vi "InstrumentSetup.vi"() -> ()   [LabVIEW 2019, in "InstrControl.lvclass"]
uses:
  InstrControl.lvclass
  SupplyControl/Keithley 236 & 237/KE236.lvclass
  SupplyControl/Keithley 6517/KE6517.lvclass
  SupplyControl/Keithley 2410/KE2410.lvclass
  SupplyControl/Keithley 487/KE487.lvclass
  ArduinoControl/ArduinoControl.lvclass
  MultimeterControl/Keithley 2000/KE2000.lvclass
  LCRControl/WK6440B/WK6440B.lvclass
  Switching/Pickering/Pickering.lvclass
  LCRControl/WK6425/WK6425.lvclass
  Switching/Keithley 3706A/KE3706A.lvclass
  Switching/LXIPXISwitching/LXIPXISwitching.lvclass
panel:
  in  "LXI/PXI Configurations":T1={"MUX"="1", "Matrix"="4", "Breadboard"="5", "LXIPXI Switching"=refnum, "MUX PN"="40-635-108", "Matrix  PN"="40-332-002", "Breadboard PN"="40-220A-501-S6", "MUX ID"="1", "Matrix ID"="4", "Breadboard ID"="5"}
  in  "Keithley 3706A Configurations":T2={"Mux1 slot"="1", "Mux2 slot"="2", "KE3706A"=refnum}
  in  "Keithley 487_2 Configurations":T3 {"Range:" items=["Autorange", "2nA", "20nA", "200nA", "2 microAmp", "20 microAmp", "200 microAmp", "2 milliAmp"]; "Compliance" items=["20µA", "2mA"]}
  in  "Instrument addresses":T4={"KE 2410"={"Instrument name"="Keithley 2410", "address"="GPIB0::16::INSTR", "Instrument type"=0}, "KE 6517"={"Instrument name"="Keithley 6517", "address"="", "Instrument type"=0}, "KE 487"={"Instrument name"="Keithley 487", "address"="", "Instrument type"=0}, "KE 236"={"Instrument name"="Keithley 236", "address"="", "Instrument type"=0}, "WK 6440B"={"Instrument name"="WayneKerr 6440B", "address"="GPIB0::6::INSTR", "Instrument type"=1}, "WK 6425"={"Instrument name"="WayneKerr 6425", "address"="", "Instrument type"=1}, "Pickering Matrix"={"Instrument name"="Pickering Matrix", "address"="GPIB0::10::INSTR", "Instrument type"=3}, "KE 2000"={"Instrument name"="Keithley 2000", "address"="GPIB0::19::INSTR", "Instrument type"=2}, "KE3706A Switching"={"Instrument name"="KE3706A", "address"="GPIB0::11::INSTR", "Instrument type"=3}} {"KE3706A Switching"."Instrument type" items=["Supply", "LCR", "Multimeter", "Switching"]; "KE 2000"."Instrument type" items=["Supply", "LCR", "Multimeter", "Switching"]; "Pickering Matrix"."Instrument type" items=["Supply", "LCR", "Multimeter", "Switching"]; "WK 6425"."Instrument type" items=["Supply", "LCR", "Multimeter", "Switching"]; "WK 6440B"."Instrument type" items=["Supply", "LCR", "Multimeter", "Switching"]; "KE 236"."Instrument type" items=["Supply", "LCR", "Multimeter", "Switching"]; "KE 487"."Instrument type" items=["Supply", "LCR", "Multimeter", "Switching"]; "KE 6517"."Instrument type" items=["Supply", "LCR", "Multimeter", "Switching"]; "KE 2410"."Instrument type" items=["Supply", "LCR", "Multimeter", "Switching"]}
  in  "WayneKerr 6425 Configurations":T5={"RC Configuration"=0, "AC amplitude [V]"=0.1, "AC frequency [Hz]"=1000, "WK6425"=refnum} {"RC Configuration" items=["serial", "parallel"]}
  in  "Pickering MUX & Matrix Configurations":T6={"Matrix address"="1", "Mux1 address"="4", "Mux2 address"="5", "Pickering"=refnum, "Matrix X Channels"={"Bias Supply / SMU LO"=5, "Bias Supply / SMU HI"=6, "CV Box LO"=3, "CV Box HI"=4, "CV Box LO IN"=7, "CV Box HI IN"=8, "Volt meter LO"=1, "Volt meter HI"=2, "Mux1 C1"=9, "Mux1 C2"=10, "Mux2 C1"=11, "Mux2 C2"=12}}
  in  "WayneKerr 6440B Configurations":T7={"RC Configuration"=0, "AC amplitude [V]"=0.1, "AC frequency [Hz]"=1000, "WK6440B"=refnum} {"RC Configuration" items=["serial", "parallel"]}
  in  "Keithley 2000 Configurations":T8={"Range"=0, "Range Value"=100.0, "Function"=3, "KE2000"=refnum} {"Function" items=["AC Current", "DC Current", "AC Voltage", "DC Voltage", "2W-Resistance", "4W-Resistance", "Period", "Frequency", "Temperature", "Diode", "Continuity"]; "Range Value" format="%#.2g"; "Range" items=["Auto", "Manual"]}
  in  "Arduino Configuration":T9={"VISA address"="COM24", "T sensor"=enum."SHT", "Arduino"=refnum}
  in  "Keithley 487 Configurations":T3 {"Range:" items=["Autorange", "2nA", "20nA", "200nA", "2 microAmp", "20 microAmp", "200 microAmp", "2 milliAmp"]; "Compliance" items=["20µA", "2mA"]}
  in  "Keithley 2410 Configurations":T10={"Current Limit"=0.0001, "KE2410"=refnum}
  in  "Keithley 6517 Configurations":T11={"Current Limit"=1, "KE6517"=refnum} {"Current Limit" items=["OFF", "ON"]}
  in  "Keithley 236 Configurations":T12={"current \ncompliance level"=0.0001, "compliance/\nmeasurement range (auto:0)"=6, "KE236"=refnum} {"compliance/\nmeasurement range (auto:0)" items=["auto / auto", "1 nA / 1.1 V", "10 nA / 11 V", "100 nA / 110 V", "0.001 mA / 110 V", "0.01 mA / 110 V", "0.1 mA / 110 V", "1 mA / 110 V", "10 mA / 110 V", "100 mA / 110 V"]; "current \ncompliance level" format="%.4f"}
  in  "Default GPIB addresses":T13={"KE 487"="22", "KE 6517"="27", "WK 6425"="17", "KE 236"="16", "HP 4263B"="18", "KE 2000"="19", "KE 2410"="24", "WK 6440B"="23", "Matrix"="10"}
  # "PROPERTY CLUSTERS + DEFAULT VALUES FOR INSTRUMENT SETUP"
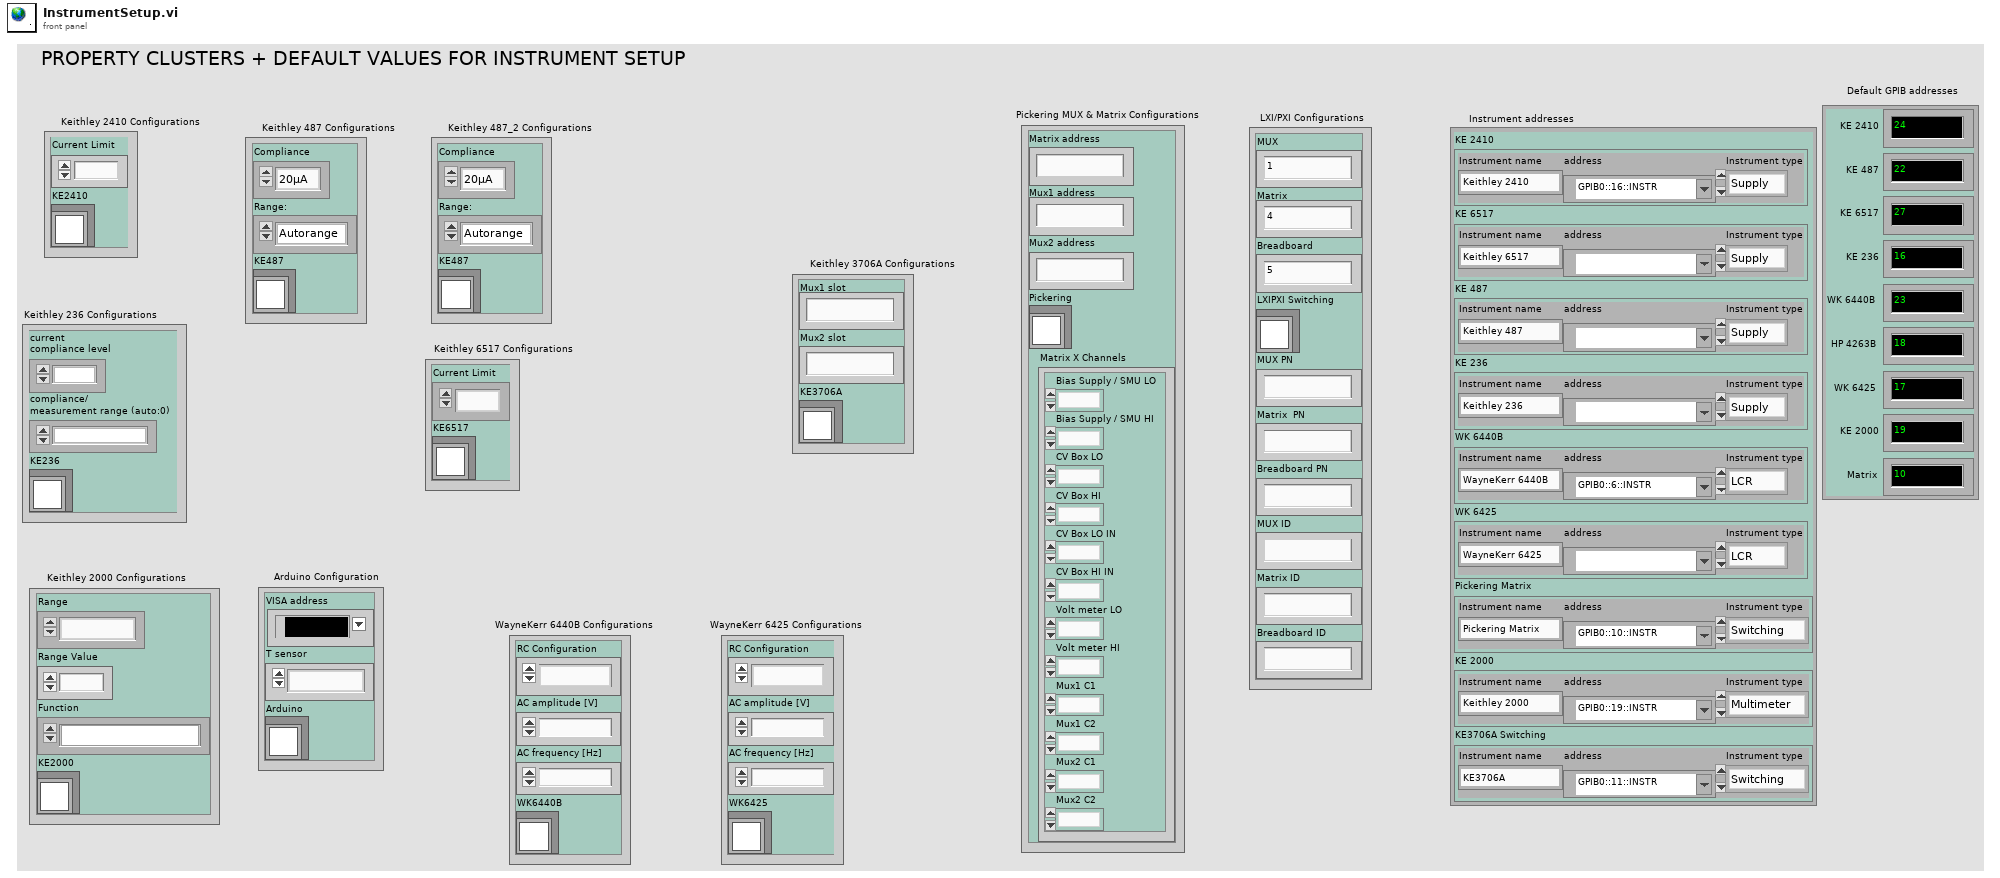
[diagram p1: front panel]
types:
  T1 = cluster{"MUX":string, "Matrix":string, "Breadboard":string, "LXIPXI Switching":refnum<class "LXIPXISwitching.lvclass">, "MUX PN":string, "Matrix  PN":string, "Breadboard PN":string, "MUX ID":string, "Matrix ID":string, "Breadboard ID":string}
  T2 = cluster{"Mux1 slot":string, "Mux2 slot":string, "KE3706A":refnum<class "KE3706A.lvclass">}
  T3 = cluster{"Compliance":u16, "Range:":u16, "KE487":refnum<class "KE487.lvclass">}
  T4 = cluster{"KE 2410":cluster{"Instrument name":string, "address":refnum<visa-resource-name>, "Instrument type":u16}, "KE 6517":cluster{"Instrument name":string, "address":refnum<visa-resource-name>, "Instrument type":u16}, "KE 487":cluster{"Instrument name":string, "address":refnum<visa-resource-name>, "Instrument type":u16}, "KE 236":cluster{"Instrument name":string, "address":refnum<visa-resource-name>, "Instrument type":u16}, "WK 6440B":cluster{"Instrument name":string, "address":refnum<visa-resource-name>, "Instrument type":u16}, "WK 6425":cluster{"Instrument name":string, "address":refnum<visa-resource-name>, "Instrument type":u16}, "Pickering Matrix":cluster{"Instrument name":string, "address":refnum<visa-resource-name>, "Instrument type":u16}, "KE 2000":cluster{"Instrument name":string, "address":refnum<visa-resource-name>, "Instrument type":u16}, "KE3706A Switching":cluster{"Instrument name":string, "address":refnum<visa-resource-name>, "Instrument type":u16}}
  T5 = cluster{"RC Configuration":u16, "AC amplitude [V]":dbl, "AC frequency [Hz]":i32, "WK6425":refnum<class "WK6425.lvclass">}
  T6 = cluster{"Matrix address":string, "Mux1 address":string, "Mux2 address":string, "Pickering":refnum<class "Pickering.lvclass">, "Matrix X Channels":cluster{"Bias Supply / SMU LO":i32, "Bias Supply / SMU HI":i32, "CV Box LO":i32, "CV Box HI":i32, "CV Box LO IN":i32, "CV Box HI IN":i32, "Volt meter LO":i32, "Volt meter HI":i32, "Mux1 C1":i32, "Mux1 C2":i32, "Mux2 C1":i32, "Mux2 C2":i32}}
  T7 = cluster{"RC Configuration":u16, "AC amplitude [V]":dbl, "AC frequency [Hz]":i32, "WK6440B":refnum<class "WK6440B.lvclass">}
  T8 = cluster{"Range":u16, "Range Value":dbl, "Function":u16, "KE2000":refnum<class "KE2000.lvclass">}
  T9 = cluster{"VISA address":refnum<visa-resource-name>, "T sensor":enum16{"SHT", "DS"}, "Arduino":refnum<class "ArduinoControl.lvclass">}
  T10 = cluster{"Current Limit":sgl, "KE2410":refnum<class "KE2410.lvclass">}
  T11 = cluster{"Current Limit":u16, "KE6517":refnum<class "KE6517.lvclass">}
  T12 = cluster{"current \ncompliance level":dbl, "compliance/\nmeasurement range (auto:0)":u16, "KE236":refnum<class "KE236.lvclass">}
  T13 = cluster{"KE 487":string, "KE 6517":string, "WK 6425":string, "KE 236":string, "HP 4263B":string, "KE 2000":string, "KE 2410":string, "WK 6440B":string, "Matrix":string}
diagram:
